vi "LoadClassFromName_core.vi"(7 "ClassTemplate":refnum<class>, 8 "error in (no error)":errorcluster, 9 "AdditionalData":variant, 10 "Class":string, 11 "DLMapper in":refnum<class "ClassLoader.lvclass">) -> (0 "error out":errorcluster, 2 "Class":refnum<class>, 3 "DLMapper out":refnum<class "ClassLoader.lvclass">)   [LabVIEW 2020, in "ClassLoader.lvlib" / "ClassLoader.lvclass"]
uses:
  ClassLoader.lvclass
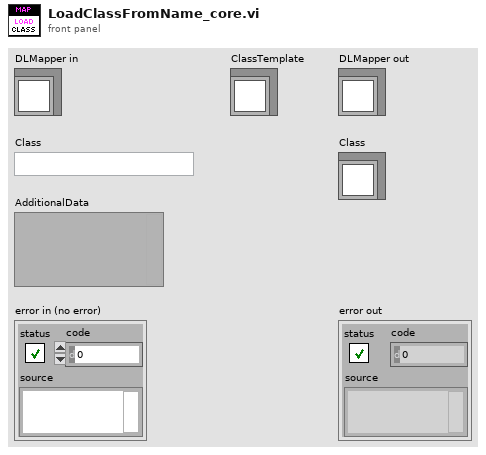
[diagram p1: front panel]
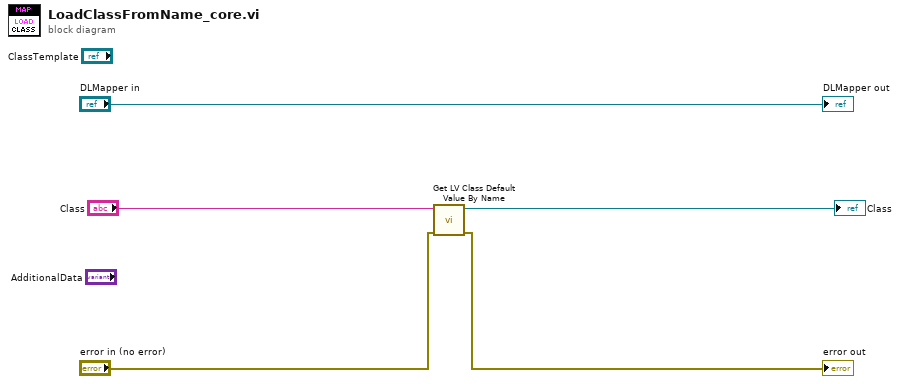
[diagram p0: block diagram]
diagram:
  n1 = call <vilib>:"Get LV Class Default Value By Name.vi"("error in (no error)"="error in (no error)", "class name"="Class") -> ("error out"=→"error out":errorcluster, "object"=→"Class":refnum<class>)  [unwired: 8 in]
  "DLMapper out" <- "DLMapper in"
